vi "brick_break_game.vi"() -> (2 "Score":i32)   [LabVIEW 2014]
uses:
  <vilib>/Utility/miscctls.llb/LVPositionTypeDef.ctl
  <vilib>/Utility/miscctls.llb/LVBoundsTypeDef.ctl
panel:
  in  "ball":bool=TRUE
  in  "ball out":u32(colorbox)=16711680
  in  "ball in":u32(colorbox)=16711680
  out "xSpeedUp":bool
  out "ySpeedUp":bool
  in  "game string":string="Game Over"
  out "x speed up":string
  out "y speed up":string
  in  "Level":i32=1
  in  "game states":T1(ring)
  out "over":bool
  out "pass time":dbl
  in  "start":bool
  out "start timer":u32
  in  "ball init pos":cluster{i32, i32}
  out "brick status":bool[](array[boolean])
  out "bricks left":i32
  out "hit block":i32
  out "y hit detec":bool[][](array[boolean])
  out "y hitbox pos":i32[][](array[numeric])
  out "x hitbox pos":i32[][](array[numeric])
  out "ball size":i32
  in  "Brick 7":u32(colorbox)
  in  "Brick 6":u32(colorbox)
  in  "Brick 0":u32(colorbox)
  in  "Brick 5":u32(colorbox)
  in  "Brick 4":u32(colorbox)
  in  "Brick 3":u32(colorbox)
  in  "Brick 2":u32(colorbox)
  in  "Brick 1":u32(colorbox)
  out "brick pos":i32[][](array[numeric])
  in  "y scale":i32=2
  in  "x scale":i32=2
  in  "brick size":cluster{"width":i32, "hight":i32}={"width"=50, "hight"=20}
  in  "Slide":u8(slide)=100 scale=0.0..100.0
  out "x hit detec":bool[][](array[boolean])
  in  "backgound":T2={"width"=400, "hight"=300, "position"=[0, 0]}
  in  "background":u32(colorbox)=13816530
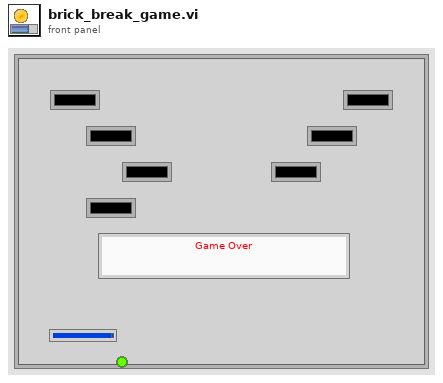
[diagram p1: front panel]
types:
  T1 = enum16{"Initialize", "Brick pos set Lv1", "Brick pos set Lv2", "Hitbox placement", "Level 1", "Level 2", "End"}
  T2 = cluster{"width":i32, "hight":i32, "position":i32[]}
  T3 = enum8{"Enabled", "Disabled", "Disabled and Grayed Out"}
  T4 = typedef "LVBoundsTypeDef.ctl" = cluster{"Width":u32, "Height":u32}
  T5 = typedef "LVPositionTypeDef.ctl" = cluster{"Left":i32, "Top":i32}
  T6 = typedef "eventvkey.ctl" = enum16{"ASCII", "Enter", "Return", "Shift", "Ctrl", "Alt", "Cmd", "Opt", "Caps", "NumLock", "Clear", "Break", "Up", "Down", "Left", "Right", "Insert", "Delete", "Home", "End", "PageUp", "PageDown", "Escape", "Help", "Pause", "ScrollLock", "F1", "F2", "F3", "F4", "F5", "F6", "F7", "F8", "F9", "F10", "F11", "F12", "F13", "F14", "F15", "F16", "F17", "F18", "F19", "F20", "F21", "F22", "F23", "F24", "Play", "VolumeUp", "VolumeDown", "Mute", "Two Byte Char"}
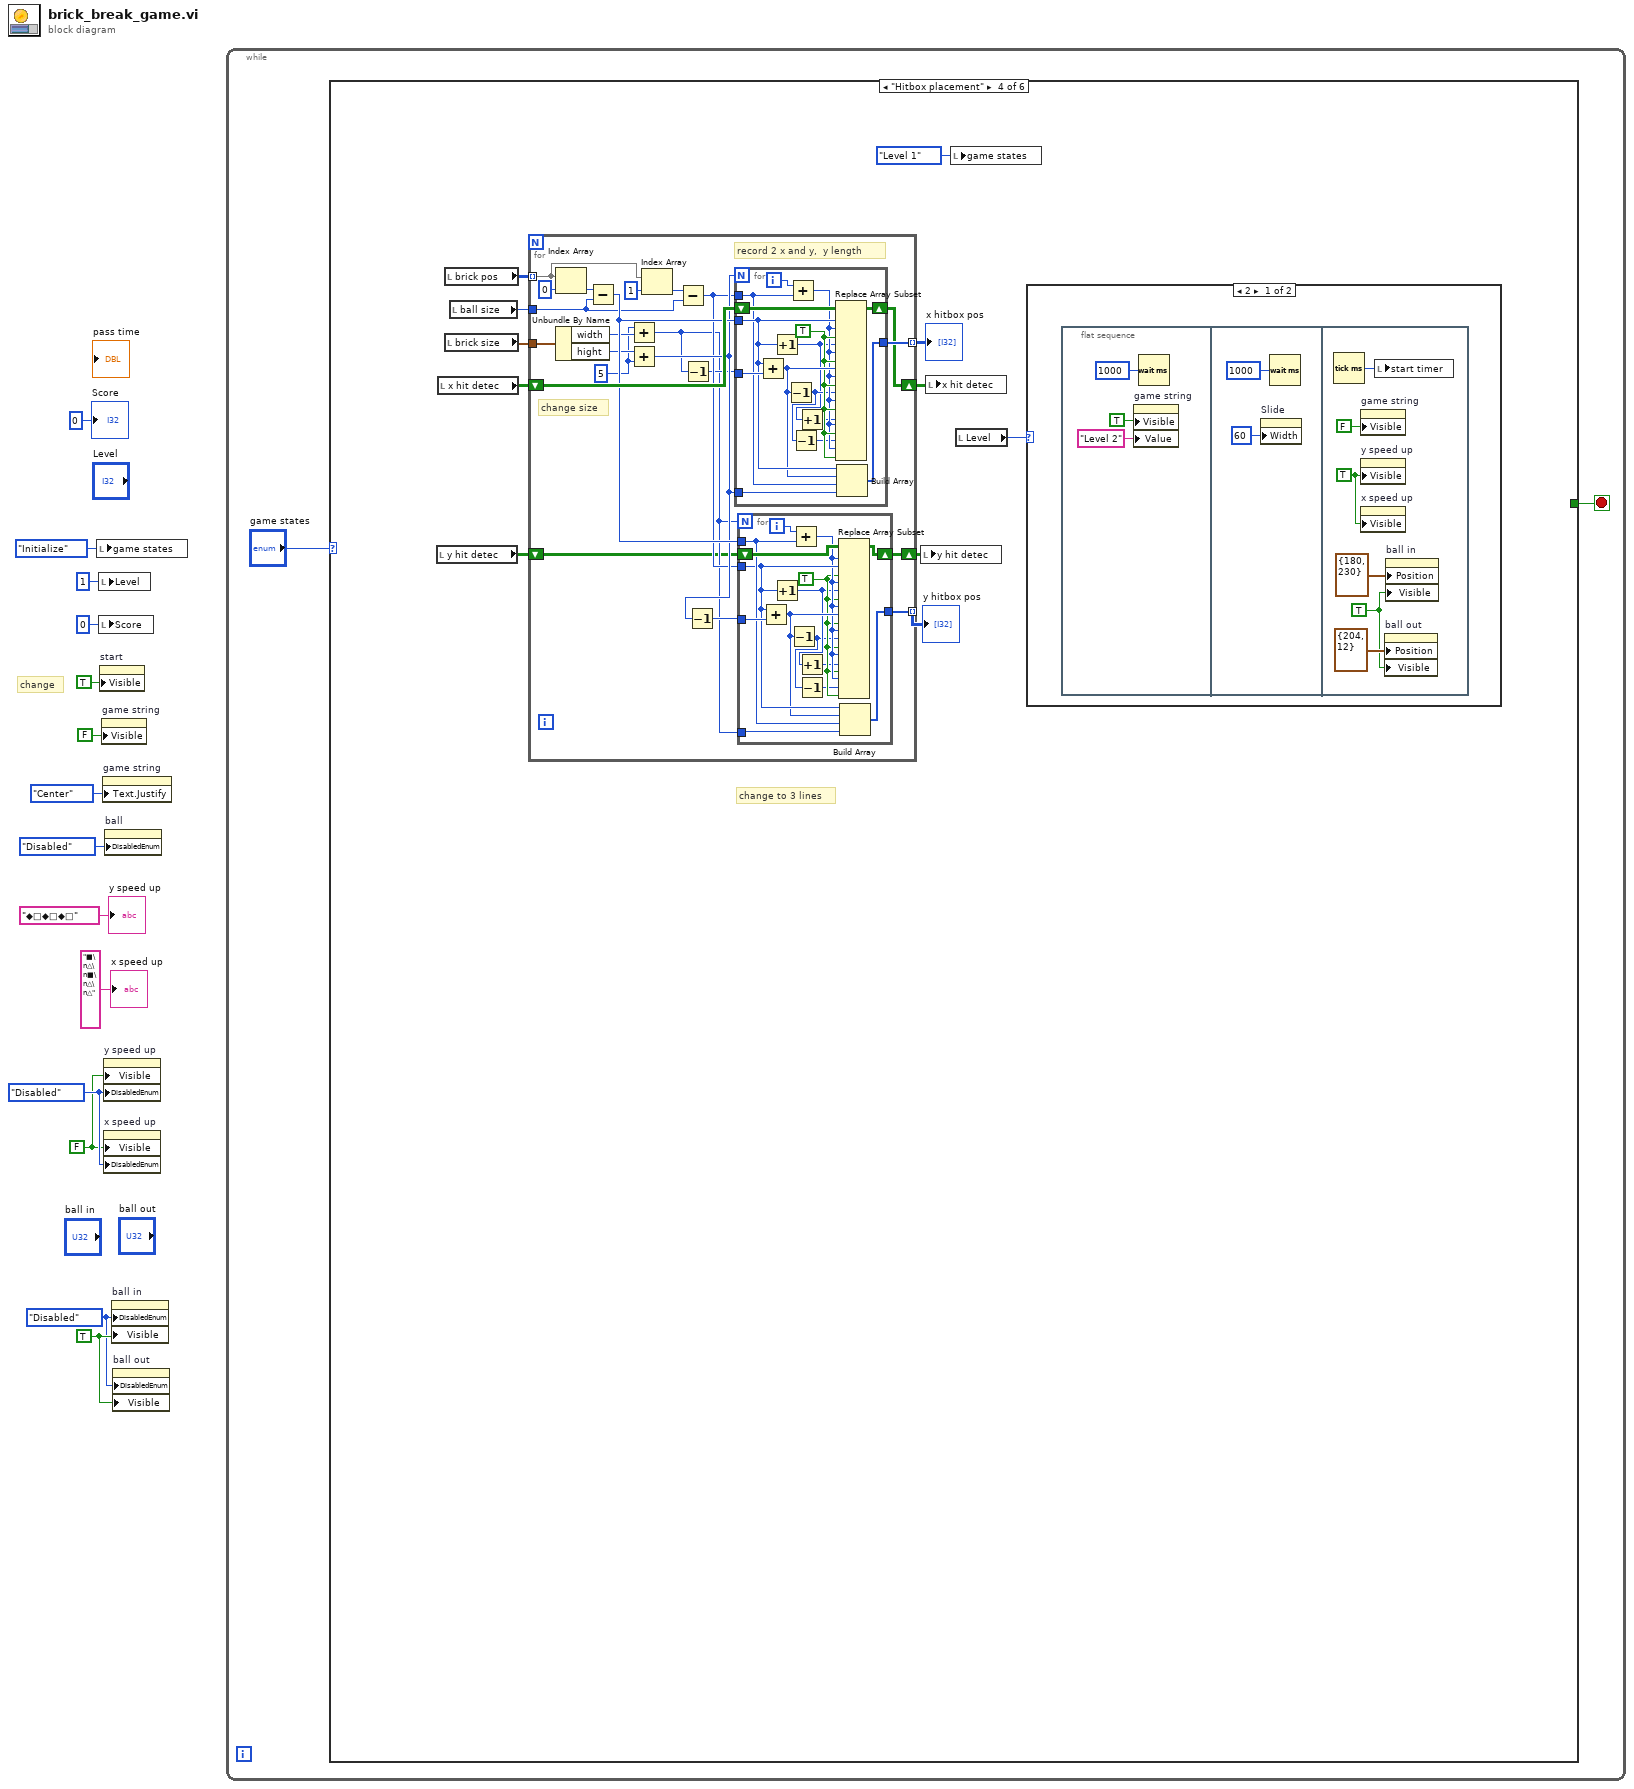
[diagram p0: block diagram]
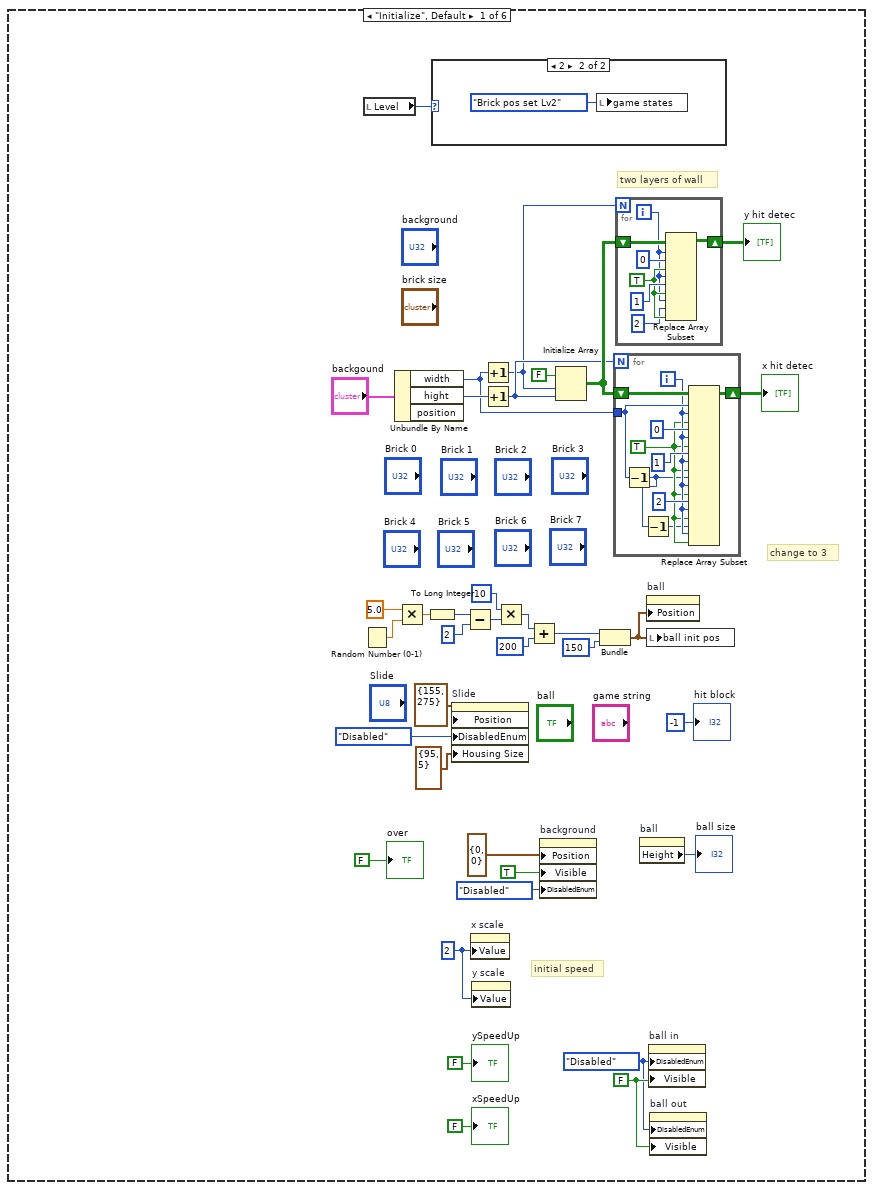
[diagram p2: hidden frame]
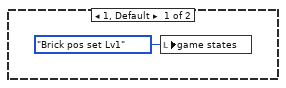
[diagram p3: hidden frame]
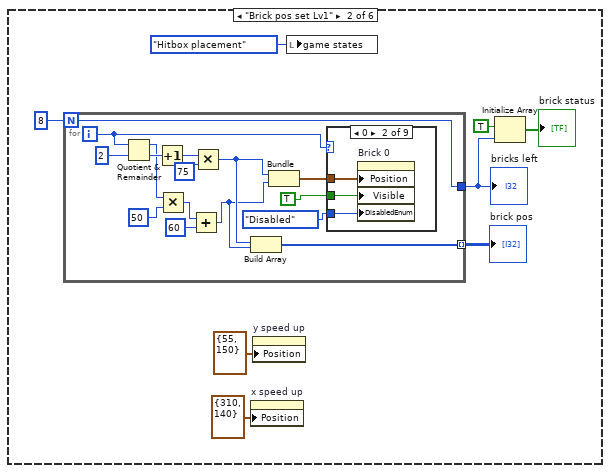
[diagram p4: hidden frame]
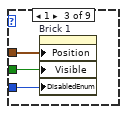
[diagram p6: hidden frame]
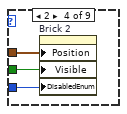
[diagram p7: hidden frame]
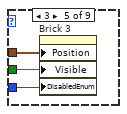
[diagram p8: hidden frame]
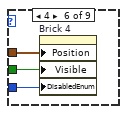
[diagram p9: hidden frame]
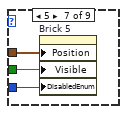
[diagram p10: hidden frame]
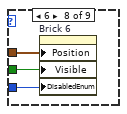
[diagram p11: hidden frame]
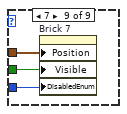
[diagram p12: hidden frame]
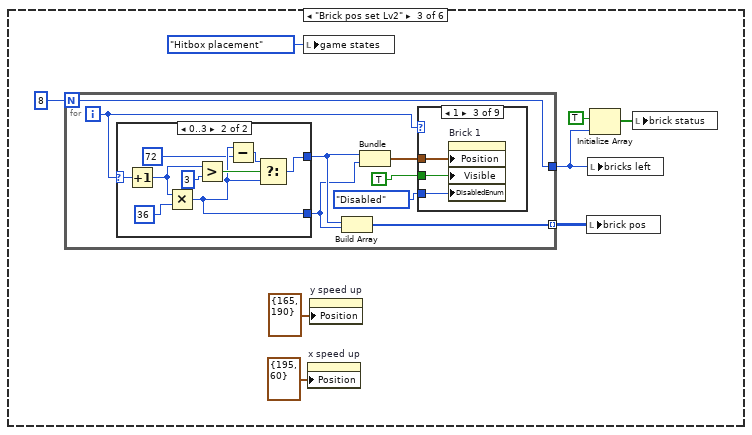
[diagram p13: hidden frame]
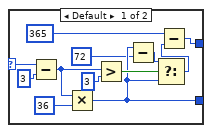
[diagram p14: hidden frame]
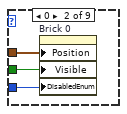
[diagram p16: hidden frame]
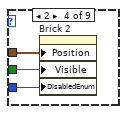
[diagram p17: hidden frame]
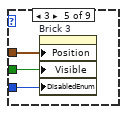
[diagram p18: hidden frame]
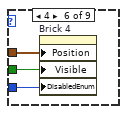
[diagram p19: hidden frame]
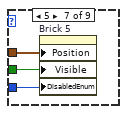
[diagram p20: hidden frame]
diagram:
  w2 = TRUE ("Visible")
  w1 = T3."Disabled" ("Disabled")
  w4 = T3."Disabled" ("Disabled")
  w3 = FALSE ("Visible")
  # "change"
  n1 = local write "game states"(T1."Initialize" ("game states")) -> ()
  n2 = local write "Level"(1 ("Level")) -> ()
  n3 = local write "Score"(0 ("Score")) -> ()
  n4 = property on="start" class="Bool"("Visible"=TRUE) -> ()  [unwired: 2 in, 2 out]
  n5 = property on="game string" class="Str"("Visible"=FALSE) -> ()  [unwired: 2 in, 2 out]
  n6 = property on="game string" class="Str"("Text.Justify"=enum16{"Left", "Center", "Right"}."Center" ("Text.Justification")) -> ()  [unwired: 2 in, 2 out]
  n7 = property on="y speed up" class="Str"("Visible"=w3, "DisabledEnum"=w4) -> ()  [unwired: 2 in, 2 out]
  n8 = property on="x speed up" class="Str"("Visible"=w3, "DisabledEnum"=w4) -> ()  [unwired: 2 in, 2 out]
  n9 = property on="ball" class="Bool (strict)"("DisabledEnum"=T3."Disabled" ("Disabled")) -> ()  [unwired: 2 in, 2 out]
  n10 = property on="ball in" class="ColBox"("DisabledEnum"=w1, "Visible"=w2) -> ()  [unwired: 2 in, 2 out]
  n11 = property on="ball out" class="ColBox"("DisabledEnum"=w1, "Visible"=w2) -> ()  [unwired: 2 in, 2 out]
  n12 = while {
    stop <- w15 stop-if-true
    n13 = case shown="\"Hitbox placement\"" "game states" {
      tunnel: [_ _ _ _ _ w845] -> w15
      frame "Initialize", Default {
        w18 = FALSE ("Visible")
        w17 = T3."Disabled" ("Disabled")
        w21 = 2 ("x scale")
        # "initial speed"
        # "change to 3"
        # "two layers of wall"
        n14 = Random Number (0-1)() -> (number: 0 to 1=w38:dbl)
        n15 = local read "Level"() -> (w23:i32)
        n16 = Unbundle By Name("backgound") -> ("width"=w46:i32, "hight"=w48:i32)  [unwired: 1 out]
        n17 = Multiply(x=5.0, y=w38) -> (x*y=w36:dbl)
        n18 = To Long Integer(number=w36) -> (32bit integer=w35:i32)
        n19 = case shown="2" w23 {
          frame 1, Default {
            n20 = local write "game states"(T1."Brick pos set Lv1" ("game states")) -> ()
          }
          frame 2 {
            n21 = local write "game states"(T1."Brick pos set Lv2" ("game states")) -> ()
          }
        }
        n22 = property on="Slide" class="Slide (strict)"("Position"=T5 {"Left"=155, "Top"=275}, "DisabledEnum"=T3."Disabled" ("Disabled"), "Housing Size"=T4 {"Width"=95, "Height"=5}) -> ()  [unwired: 2 in, 2 out]
        n23 = Subtract(x=w35, y=2) -> (x-y=w30:i32)
        n24 = property on="x scale" class="DigNum (strict)"("Value"=w21) -> ()  [unwired: 2 in, 2 out]
        n25 = property on="y scale" class="DigNum (strict)"("Value"=w21) -> ()  [unwired: 2 in, 2 out]
        n26 = Increment(x=w46) -> (x+1=w47:i32)
        n27 = Increment(x=w48) -> (x+1=w49:i32)
        n28 = Multiply(x=10 ("y"), y=w30) -> (x*y=w33:i32)
        n29 = Add(x=w33, y=200) -> (x+y=w31:i32)
        n30 = property on="background" class="ColBox"("Position"=T5 {"Left"=0, "Top"=0}, "Visible"=TRUE, "DisabledEnum"=T3."Disabled" ("Disabled")) -> ()  [unwired: 2 in, 2 out]
        n31 = Initialize Array(FALSE, w47, w49) -> (w50:bool[][])
        n32 = Bundle(w31, 150) -> (w40:cluster{i32, i32})  [unwired: 1 in]
        n33 = for {
          N: w49 -> [_]
          shift-right: [w70] -> w51
          shift-left: w50 -> [w71]
          tunnel: w46 -> [w68]
          i -> [w65]
          w64 = TRUE
          n34 = Decrement(x=w68) -> (x-1=w63:i32)
          n35 = Decrement(x=w63) -> (x-1=w62:i32)
          n36 = Replace Array Subset(array=w71, new element #1=w64, index (row) #1=w68, index (col) #1=w65, new element #2=w64, index (row) #2=0, index (col) #2=w65, new element #3=w64, index (row) #3=1 ("disabled index (row)"), index (col) #3=w65, new element #4=w64, index (row) #4=w63, index (col) #4=w65, new element #5=w64, index (row) #5=2, index (col) #5=w65, new element #6=w64, index (row) #6=w62, index (col) #6=w65) -> (w70:bool[][])
        }
        "x hit detec" <- w51
        n37 = for {
          N: w47 -> [_]
          shift-right: [w60] -> w52
          shift-left: w50 -> [w61]
          i -> [w56]
          w57 = TRUE
          n38 = Replace Array Subset(array=w61, new element #1=w57, index (row) #1=w56, index (col) #1=0 ("index (col)"), new element #2=w57, index (row) #2=w56, index (col) #2=1 ("disabled index (col)"), new element #3=w57, index (row) #3=w56, index (col) #3=2) -> (w60:bool[][])
        }
        "y hit detec" <- w52
        n39 = property on="ball" class="Bool (strict)"() -> ("Height"=→"ball size":u32)  [unwired: 2 in, 2 out]
        n40 = property on="ball" class="Bool (strict)"("Position"=w40) -> ()  [unwired: 2 in, 2 out]
        n41 = local write "ball init pos"(w40) -> ()
        n42 = property on="ball in" class="ColBox"("DisabledEnum"=w17, "Visible"=w18) -> ()  [unwired: 2 in, 2 out]
        n43 = property on="ball out" class="ColBox"("DisabledEnum"=w17, "Visible"=w18) -> ()  [unwired: 2 in, 2 out]
        "hit block" <- -1 ("hit block")
        "over" <- FALSE ("over")
        "ySpeedUp" <- FALSE ("ySpeedUp")
        "xSpeedUp" <- FALSE ("xSpeedUp")
      }
      frame "Brick pos set Lv1" {
        n44 = for {
          N: 8 -> [w80]
          tunnel: [w86] -> w78 mode=indexing
          tunnel: [w80] -> w76
          i -> [w81]
          n45 = Quotient & Remainder(x=w81, y=2) -> (x-y*floor(x/y)=w88:i32, floor(x/y)=w93:i32)
          n46 = Increment(x=w93) -> (x+1=w92:i32)
          n47 = Multiply(x=w88, y=50) -> (x*y=w85:i32)
          n48 = Add(x=w85, y=60) -> (x+y=w84:i32)
          n49 = Multiply(x=w92, y=75) -> (x*y=w87:i32)
          n50 = Build Array(w87, w84) -> (w86:i32[])
          n51 = Bundle(w87, w84) -> (w89:cluster{i32, i32})  [unwired: 1 in]
          n52 = case shown="0" w81 {
            tunnel: TRUE -> [_ w98 w101 w104 w107 w110 w113 w115 w119]
            tunnel: w89 -> [_ w97 w100 w103 w106 w109 w112 w116 w118]
            tunnel: T3."Disabled" ("Disabled") -> [_ w96 w99 w102 w105 w108 w111 w114 w117]
            frame Default {
            }
            frame 0 {
              n53 = property on="Brick 0" class="ColBox"("Position"=w97, "Visible"=w98, "DisabledEnum"=w96) -> ()  [unwired: 2 in, 2 out]
            }
            frame 1 {
              n54 = property on="Brick 1" class="ColBox"("Position"=w100, "Visible"=w101, "DisabledEnum"=w99) -> ()  [unwired: 2 in, 2 out]
            }
            frame 2 {
              n55 = property on="Brick 2" class="ColBox"("Position"=w103, "Visible"=w104, "DisabledEnum"=w102) -> ()  [unwired: 2 in, 2 out]
            }
            frame 3 {
              n56 = property on="Brick 3" class="ColBox"("Position"=w106, "Visible"=w107, "DisabledEnum"=w105) -> ()  [unwired: 2 in, 2 out]
            }
            frame 4 {
              n57 = property on="Brick 4" class="ColBox"("Position"=w109, "Visible"=w110, "DisabledEnum"=w108) -> ()  [unwired: 2 in, 2 out]
            }
            frame 5 {
              n58 = property on="Brick 5" class="ColBox"("Position"=w112, "Visible"=w113, "DisabledEnum"=w111) -> ()  [unwired: 2 in, 2 out]
            }
            frame 6 {
              n59 = property on="Brick 6" class="ColBox"("Position"=w116, "Visible"=w115, "DisabledEnum"=w114) -> ()  [unwired: 2 in, 2 out]
            }
            frame 7 {
              n60 = property on="Brick 7" class="ColBox"("Position"=w118, "Visible"=w119, "DisabledEnum"=w117) -> ()  [unwired: 2 in, 2 out]
            }
          }
        }
        "brick pos" <- w78
        "bricks left" <- w76
        n61 = property on="x speed up" class="Str"("Position"=T5 {"Left"=310, "Top"=140}) -> ()  [unwired: 2 in, 2 out]
        n62 = property on="y speed up" class="Str"("Position"=T5 {"Left"=55, "Top"=150}) -> ()  [unwired: 2 in, 2 out]
        n63 = local write "game states"(T1."Hitbox placement" ("game states")) -> ()
        n64 = Initialize Array(TRUE, w76) -> (→"brick status":bool[])
      }
      frame "Brick pos set Lv2" {
        n65 = for {
          N: 8 -> [w131]
          tunnel: [w133] -> w123 mode=indexing
          tunnel: [w131] -> w122
          i -> [w128]
          n66 = case shown="0..3" w128 {
            selector: w128 -> [w147 w156]
            tunnel: [w137 w149] -> w130
            tunnel: [w140 w152] -> w129
            frame Default {
              n67 = Subtract(x=w147, y=3) -> (x-y=w141:i32)
              n68 = Multiply(x=w141, y=36) -> (x*y=w140:i32)
              n69 = Greater?(x=w141, y=3) -> (0:w143:bool)
              n70 = Subtract(x=w140, y=72) -> (x-y=w142:i32)
              n71 = Select(t=w142, s=w143, f=w140) -> (s? t:f=w138:i32)
              n72 = Subtract(x=365, y=w138) -> (x-y=w137:i32)
            }
            frame 0..3 {
              n73 = Increment(x=w156) -> (x+1=w155:i32)
              n74 = Multiply(x=w155, y=36) -> (x*y=w152:i32)
              n75 = Greater?(x=w155, y=3) -> (0:w153:bool)
              n76 = Subtract(x=w152, y=72) -> (x-y=w150:i32)
              n77 = Select(t=w150, s=w153, f=w152) -> (s? t:f=w149:i32)
            }
          }
          n78 = Build Array(w130, w129) -> (w133:i32[])
          n79 = Bundle(w130, w129) -> (w134:cluster{i32, i32})  [unwired: 1 in]
          n80 = case shown="1" w128 {
            tunnel: TRUE -> [_ w159 w162 w165 w168 w171 w174 w176 w180]
            tunnel: w134 -> [_ w158 w161 w164 w167 w170 w173 w177 w179]
            tunnel: T3."Disabled" ("Disabled") -> [_ w157 w160 w163 w166 w169 w172 w175 w178]
            frame Default {
            }
            frame 0 {
              n81 = property on="Brick 0" class="ColBox"("Position"=w158, "Visible"=w159, "DisabledEnum"=w157) -> ()  [unwired: 2 in, 2 out]
            }
            frame 1 {
              n82 = property on="Brick 1" class="ColBox"("Position"=w161, "Visible"=w162, "DisabledEnum"=w160) -> ()  [unwired: 2 in, 2 out]
            }
            frame 2 {
              n83 = property on="Brick 2" class="ColBox"("Position"=w164, "Visible"=w165, "DisabledEnum"=w163) -> ()  [unwired: 2 in, 2 out]
            }
            frame 3 {
              n84 = property on="Brick 3" class="ColBox"("Position"=w167, "Visible"=w168, "DisabledEnum"=w166) -> ()  [unwired: 2 in, 2 out]
            }
            frame 4 {
              n85 = property on="Brick 4" class="ColBox"("Position"=w170, "Visible"=w171, "DisabledEnum"=w169) -> ()  [unwired: 2 in, 2 out]
            }
            frame 5 {
              n86 = property on="Brick 5" class="ColBox"("Position"=w173, "Visible"=w174, "DisabledEnum"=w172) -> ()  [unwired: 2 in, 2 out]
            }
            frame 6 {
              n87 = property on="Brick 6" class="ColBox"("Position"=w177, "Visible"=w176, "DisabledEnum"=w175) -> ()  [unwired: 2 in, 2 out]
            }
            frame 7 {
              n88 = property on="Brick 7" class="ColBox"("Position"=w179, "Visible"=w180, "DisabledEnum"=w178) -> ()  [unwired: 2 in, 2 out]
            }
          }
        }
        n89 = local write "game states"(T1."Hitbox placement" ("game states")) -> ()
        n90 = property on="x speed up" class="Str"("Position"=T5 {"Left"=195, "Top"=60}) -> ()  [unwired: 2 in, 2 out]
        n91 = property on="y speed up" class="Str"("Position"=T5 {"Left"=165, "Top"=190}) -> ()  [unwired: 2 in, 2 out]
        n92 = local write "brick pos"(w123) -> ()
        n93 = local write "bricks left"(w122) -> ()
        n94 = Initialize Array(TRUE, w122) -> (w125:bool[])
        n95 = local write "brick status"(w125) -> ()
      }
      frame "Hitbox placement" {
        # "change to 3 lines"
        n96 = local read "y hit detec"() -> (w190:bool[][])
        n97 = local read "x hit detec"() -> (w184:bool[][])
        n98 = local read "brick pos"() -> (w183:i32[][])
        n99 = local read "brick size"() -> (w185:cluster{"width":i32, "hight":i32})
        n100 = local read "ball size"() -> (w186:i32)
        n101 = for {
          tunnel: w183 -> [w236] mode=indexing
          tunnel: w185 -> [w239]
          tunnel: w186 -> [w227]
          shift-right: [w221] -> w187
          shift-left: w184 -> [w233]
          tunnel: [w232] -> w188 mode=indexing
          tunnel: [w230] -> w189 mode=indexing
          shift-right: [w219] -> w191
          shift-left: w190 -> [w220]
          w218 = 5
          # "change size"
          # "record 2 x and y,  y length"
          n102 = Index Array(array=w236, index=0) -> (element=w235:i32)
          n103 = Unbundle By Name(w239) -> ("width"=w229:i32, "hight"=w228:i32)
          n104 = Subtract(x=w235, y=w227) -> (x-y=w231:i32)
          n105 = Add(x=w218, y=w229) -> (x+y=w222:i32)
          n106 = Add(x=w228, y=w218) -> (x+y=w226:i32)
          n107 = Index Array(array=w236, index=1) -> (element=w234:i32)
          n108 = Subtract(x=w234, y=w227) -> (x-y=w224:i32)
          n109 = Decrement(x=w222) -> (x-1=w223:i32)
          n110 = Decrement(x=w226) -> (x-1=w225:i32)
          n111 = for {
            N: w226 -> [_]
            tunnel: w231 -> [w265]
            tunnel: w224 -> [w261]
            tunnel: w223 -> [w267]
            shift-right: [w266] -> w221
            shift-left: w233 -> [w269]
            tunnel: [w264] -> w232
            tunnel: w226 -> [w262]
            i -> [w268]
            w260 = TRUE
            n112 = Add(x=w265, y=w267) -> (x+y=w263:i32)
            n113 = Increment(x=w265) -> (x+1=w255:i32)
            n114 = Decrement(x=w263) -> (x-1=w257:i32)
            n115 = Add(x=w268, y=w261) -> (x+y=w259:i32)
            n116 = Decrement(x=w257) -> (x-1=w258:i32)
            n117 = Increment(x=w255) -> (x+1=w256:i32)
            n118 = Replace Array Subset(array=w269, new element #1=w260, index (row) #1=w265, index (col) #1=w259, new element #2=w260, index (row) #2=w255, index (col) #2=w259, new element #3=w260, index (row) #3=w263, index (col) #3=w259, new element #4=w260, index (row) #4=w257, index (col) #4=w259, new element #5=w260, index (row) #5=w256, index (col) #5=w259, new element #6=w260, index (row) #6=w258, index (col) #6=w259) -> (w266:bool[][])
            n119 = Build Array(w265, w263, w261, w262) -> (w264:i32[])
          }
          n120 = for {
            N: w222 -> [_]
            tunnel: w224 -> [w247]
            tunnel: w231 -> [w248]
            tunnel: w225 -> [w252]
            shift-right: [w251] -> w219
            shift-left: w220 -> [w254]
            tunnel: [w250] -> w230
            tunnel: w222 -> [w249]
            i -> [w253]
            w244 = TRUE
            n121 = Add(x=w247, y=w252) -> (x+y=w246:i32)
            n122 = Increment(x=w247) -> (x+1=w242:i32)
            n123 = Decrement(x=w246) -> (x-1=w240:i32)
            n124 = Add(x=w253, y=w248) -> (x+y=w245:i32)
            n125 = Increment(x=w242) -> (x+1=w243:i32)
            n126 = Decrement(x=w240) -> (x-1=w241:i32)
            n127 = Replace Array Subset(array=w254, new element #1=w244, index (row) #1=w245, index (col) #1=w247, new element #2=w244, index (row) #2=w245, index (col) #2=w242, new element #3=w244, index (row) #3=w245, index (col) #3=w246, new element #4=w244, index (row) #4=w245, index (col) #4=w240, new element #5=w244, index (row) #5=w245, index (col) #5=w243, new element #6=w244, index (row) #6=w245, index (col) #6=w241) -> (w251:bool[][])
            n128 = Build Array(w247, w246, w248, w249) -> (w250:i32[])
          }
        }
        "x hitbox pos" <- w188
        "y hitbox pos" <- w189
        n129 = local write "y hit detec"(w191) -> ()
        n130 = local write "x hit detec"(w187) -> ()
        n131 = local write "game states"(T1."Level 1" ("game states")) -> ()
        n132 = local read "Level"() -> (w182:i32)
        n133 = case shown="2" w182 {
          frame 2 {
            n134 = flat-sequence {
              frame #0 {
                n135 = property on="game string" class="Str"("Visible"=TRUE, "Value"="Level 2" ("game over")) -> ()  [unwired: 2 in, 2 out]
                n136 = Wait (ms)(milliseconds to wait=u32 1000) -> ()  [unwired: 1 out]
              }
              frame #1 {
                n137 = property on="Slide" class="Slide (strict)"("Width"=u32 60 ("Housing Size:Width")) -> ()  [unwired: 2 in, 2 out]
                n138 = Wait (ms)(milliseconds to wait=u32 1000) -> ()  [unwired: 1 out]
              }
              frame #2 {
                w198 = TRUE
                w200 = TRUE ("Visible")
                n139 = Tick Count (ms)() -> (millisecond timer value=w201:u32)
                n140 = property on="game string" class="Str"("Visible"=FALSE) -> ()  [unwired: 2 in, 2 out]
                n141 = property on="y speed up" class="Str"("Visible"=w200) -> ()  [unwired: 2 in, 2 out]
                n142 = property on="x speed up" class="Str"("Visible"=w200) -> ()  [unwired: 2 in, 2 out]
                n143 = local write "start timer"(w201) -> ()
                n144 = property on="ball out" class="ColBox"("Position"=T5 {"Left"=204, "Top"=12}, "Visible"=w198) -> ()  [unwired: 2 in, 2 out]
                n145 = property on="ball in" class="ColBox"("Position"=T5 {"Left"=180, "Top"=230}, "Visible"=w198) -> ()  [unwired: 2 in, 2 out]
              }
            }
          }
          frame 1, Default {
            n146 = while {
              stop <- w203 stop-if-true
              n147 = case shown="True" "start" {
                selector: "start" -> [w206 w207]
                tunnel: [w206 w207] -> w203
                frame False {
                }
                frame True {
                  n148 = flat-sequence {
                    frame #0 {
                      n149 = property on="start" class="Bool"("Visible"=FALSE) -> ()  [unwired: 2 in, 2 out]
                      n150 = property on="game string" class="Str"("Visible"=TRUE, "Value"="Level 1" ("game over")) -> ()  [unwired: 2 in, 2 out]
                      n151 = Wait (ms)(milliseconds to wait=u32 1000) -> ()  [unwired: 1 out]
                    }
                    frame #1 {
                      w213 = TRUE
                      w215 = TRUE ("Visible")
                      n152 = Tick Count (ms)() -> (millisecond timer value=→"start timer":u32)
                      n153 = property on="game string" class="Str"("Visible"=FALSE) -> ()  [unwired: 2 in, 2 out]
                      n154 = property on="ball out" class="ColBox"("Position"=T5 {"Left"=204, "Top"=12}, "Visible"=w213) -> ()  [unwired: 2 in, 2 out]
                      n155 = property on="ball in" class="ColBox"("Position"=T5 {"Left"=180, "Top"=230}, "Visible"=w213) -> ()  [unwired: 2 in, 2 out]
                      n156 = property on="y speed up" class="Str"("Visible"=w215) -> ()  [unwired: 2 in, 2 out]
                      n157 = property on="x speed up" class="Str"("Visible"=w215) -> ()  [unwired: 2 in, 2 out]
                    }
                  }
                }
              }
              n158 = Wait Until Next ms Multiple(millisecond multiple=u32 100 ("milliseconds to wait")) -> ()  [unwired: 1 out]
            }
          }
        }
      }
      frame "Level 1" {
        # "red hole move"
        # "speed up"
        # "delete bricks"
        # "ball movements"
        # "control slide"
        n159 = local read "Level"() -> (w273:i32)
        n160 = while {
          stop <- w709 stop-if-true
          n161 = event shown="[0] \"hit block\": Value Change" {
            selector: _ -> [_ _]
            dyn-events: _ -> [_ _]
            timeout: _ -> [_ _]
            tunnel: [w713 w776] -> w709
            event "hit block": Value Change {
              n162 = event-data() -> ("NewVal"=w711:i32)  [unwired: 1 in]
              n163 = local read "brick status"() -> (w712:bool[])
              n164 = Index Array(array=w712, index=w711) -> (element=w710:bool)
              n165 = case shown="True" w710 {
                tunnel: w711 -> [_ w717]
                tunnel: [FALSE w720] -> w713
                frame False {
                }
                frame True {
                  w736 = 3 ("index")
                  w737 = 2 ("index")
                  w738 = 1 ("index")
                  w739 = 0 ("index")
                  # "change to 3"
                  n166 = local read "brick status"() -> (w718:bool[])
                  n167 = local read "x hitbox pos"() -> (w743:i32[][])
                  n168 = local read "y hitbox pos"() -> (w742:i32[][])
                  n169 = local read "bricks left"() -> (w722:i32)
                  n170 = local write "hit block"(-1 ("hit block")) -> ()
                  n171 = Decrement(x=w722) -> (x-1=w721:i32)
                  n172 = Replace Array Subset(array=w718, new element=FALSE ("new element/subarray"), index=w717) -> (w715:bool[])
                  n173 = case shown="7" w717 {
                    tunnel: FALSE -> [_ w744 w745 w746 w747 w748 w749 w750 w751]
                    frame Default {
                    }
                    frame 0 {
                      n174 = property on="Brick 0" class="ColBox"("Visible"=w744) -> ()  [unwired: 2 in, 2 out]
                    }
                    frame 1 {
                      n175 = property on="Brick 1" class="ColBox"("Visible"=w745) -> ()  [unwired: 2 in, 2 out]
                    }
                    frame 2 {
                      n176 = property on="Brick 2" class="ColBox"("Visible"=w746) -> ()  [unwired: 2 in, 2 out]
                    }
                    frame 3 {
                      n177 = property on="Brick 3" class="ColBox"("Visible"=w747) -> ()  [unwired: 2 in, 2 out]
                    }
                    frame 4 {
                      n178 = property on="Brick 4" class="ColBox"("Visible"=w748) -> ()  [unwired: 2 in, 2 out]
                    }
                    frame 5 {
                      n179 = property on="Brick 5" class="ColBox"("Visible"=w749) -> ()  [unwired: 2 in, 2 out]
                    }
                    frame 6 {
                      n180 = property on="Brick 6" class="ColBox"("Visible"=w750) -> ()  [unwired: 2 in, 2 out]
                    }
                    frame 7 {
                      n181 = property on="Brick 7" class="ColBox"("Visible"=w751) -> ()  [unwired: 2 in, 2 out]
                    }
                  }
                  n182 = Index Array(array=w743, index (row)=w717) -> (element=w741:i32[])  [unwired: 1 in]
                  n183 = Index Array(array=w742, index (row)=w717) -> (element=w740:i32[])  [unwired: 1 in]
                  n184 = Equal To 0?(x=w721) -> (x = 0?=w720:bool)
                  n185 = property on="bricks left" class="DigNum (strict)"("Val(Sgnl)"=w721) -> ()  [unwired: 2 in, 2 out]
                  n186 = local write "brick status"(w715) -> ()
                  n187 = Index Array(array=w741, index #1=w739, index #2=w738, index #3=w737, index #4=w736) -> (element #1=w733:i32, element #2=w732:i32, element #3=w731:i32, element #4=w734:i32)
                  n188 = Index Array(array=w740, index #1=w739, index #2=w738, index #3=w737, index #4=w736) -> (element #1=w727:i32, element #2=w726:i32, element #3=w725:i32, element #4=w728:i32)
                  n189 = local read "y hit detec"() -> (w729:bool[][])
                  n190 = local read "x hit detec"() -> (w735:bool[][])
                  n191 = for {
                    N: w734 -> [_]
                    shift-right: [w774] -> w730
                    shift-left: w735 -> [w775]
                    tunnel: w733 -> [w773]
                    tunnel: w732 -> [w772]
                    tunnel: w731 -> [w770]
                    i -> [w771]
                    w769 = FALSE
                    n192 = Add(x=w770, y=w771) -> (x+y=w768:i32)
                    n193 = Increment(x=w773) -> (x+1=w767:i32)
                    n194 = Decrement(x=w772) -> (x-1=w765:i32)
                    n195 = Increment(x=w767) -> (x+1=w766:i32)
                    n196 = Decrement(x=w765) -> (x-1=w764:i32)
                    n197 = Replace Array Subset(array=w775, new element #1=w769, index (row) #1=w773, index (col) #1=w768, new element #2=w769, index (row) #2=w767, index (col) #2=w768, new element #3=w769, index (row) #3=w772, index (col) #3=w768, new element #4=w769, index (row) #4=w765, index (col) #4=w768, new element #5=w769, index (row) #5=w766, index (col) #5=w768, new element #6=w769, index (row) #6=w764, index (col) #6=w768) -> (w774:bool[][])
                  }
                  n198 = for {
                    N: w728 -> [_]
                    shift-right: [w762] -> w724
                    shift-left: w729 -> [w763]
                    tunnel: w727 -> [w759]
                    tunnel: w726 -> [w758]
                    tunnel: w725 -> [w760]
                    i -> [w761]
                    w757 = FALSE
                    n199 = Add(x=w760, y=w761) -> (x+y=w756:i32)
                    n200 = Increment(x=w759) -> (x+1=w755:i32)
                    n201 = Decrement(x=w758) -> (x-1=w753:i32)
                    n202 = Increment(x=w755) -> (x+1=w754:i32)
                    n203 = Decrement(x=w753) -> (x-1=w752:i32)
                    n204 = Replace Array Subset(array=w763, new element #1=w757, index (row) #1=w756, index (col) #1=w759, new element #2=w757, index (row) #2=w756, index (col) #2=w755, new element #3=w757, index (row) #3=w756, index (col) #3=w758, new element #4=w757, index (row) #4=w756, index (col) #4=w753, new element #5=w757, index (row) #5=w756, index (col) #5=w754, new element #6=w757, index (row) #6=w756, index (col) #6=w752) -> (w762:bool[][])
                  }
                  n205 = local write "x hit detec"(w730) -> ()
                  n206 = local write "y hit detec"(w724) -> ()
                }
              }
            }
            event "over": Value Change {
              n207 = event-data() -> ("NewVal"=w776:bool)  [unwired: 1 in]
            }
          }
        }
        n208 = case shown="1, Default" w273 {
          frame 1, Default {
            w337 = FALSE
            n209 = Random Number (0-1)() -> (number: 0 to 1=w340:dbl)
            n210 = To Long Integer(number=w340) -> (32bit integer=w339:i32)
            n211 = case shown="0, Default" w339 {
              selector: w339 -> [_ w346]
              tunnel: [-1 w346] -> w344
              frame 0, Default {
              }
              frame 1 {
              }
            }
            n212 = Unbundle("ball init pos") -> (w342:i32, w343:i32)
            n213 = while {
              shift-right: [w348] -> _
              shift-left: w342 -> [w354]
              shift-right: [w347] -> _
              shift-left: w343 -> [w355]
              shift-right: [w402] -> _
              shift-left: w344 -> [w407]
              shift-right: [w392] -> _
              shift-left: 1 -> [w405]
              shift-right: [w360] -> _
              shift-left: w337 -> [w363]
              shift-right: [w357] -> _
              shift-left: w337 -> [w362]
              stop <- w394 stop-if-true
              w366 = 45
              w380 = 45
              # "init value set"
              n214 = flat-sequence {
                tunnel: w354 -> [w416]
                tunnel: w355 -> [w415]
                tunnel: [w414] -> w350
                tunnel: [w413] -> w353
                tunnel: [w412] -> w351
                frame #0 {
                  # "x"
                  # "y"
                  n215 = property on="ball in" class="ColBox"() -> ("Bounds"=w438:T4)  [unwired: 2 in, 2 out]
                  n216 = property on="ball in" class="ColBox"() -> ("Position"=w437:T5)  [unwired: 2 in, 2 out]
                  n217 = Unbundle(w438) -> ("Width"=w421:u32, "Height"=w422:u32)
                  n218 = Unbundle(w437) -> ("Left"=w430:i32, "Top"=w428:i32)
                  n219 = To Quad Integer(1:w422) -> (0:w419:i64)
                  n220 = To Quad Integer(1:w421) -> (0:w420:i64)
                  n221 = Subtract(x=w420, y=u32 10) -> (x-y=w427:i64)
                  n222 = Subtract(x=w419, y=i64 10) -> (x-y=w426:i64)
                  n223 = Subtract(x=w415, y=w428) -> (x-y=w425:i32)
                  n224 = Subtract(x=w416, y=w430) -> (x-y=w429:i32)
                  n225 = Greater?(x=w429, y=-1) -> (0:w435:bool)
                  n226 = Less?(x=w429, y=w427) -> (x < y?=w436:bool)
                  n227 = Greater Or Equal?(x=w425, y=-1) -> (x >= y?=w432:bool)
                  n228 = Less Or Equal?(x=w425, y=w426) -> (x <= y?=w431:bool)
                  n229 = And(x=w435, y=w436) -> (x .and. y?=w434:bool)
                  n230 = And(x=w432, y=w431) -> (x .and. y?=w433:bool)
                  n231 = And(x=w434, y=w433) -> (x .and. y?=w417:bool)
                  n232 = case shown="True" w417 {
                    selector: w417 -> [w439 w442]
                    tunnel: w416 -> [w441 _]
                    tunnel: w415 -> [w440 _]
                    tunnel: [w441 w444] -> w414
                    tunnel: [w440 w443] -> w413
                    tunnel: [w439 w442] -> w412
                    frame False {
                    }
                    frame True {
                      w448 = 2.0 ("y")
                      w455 = 3 ("x")
                      n233 = property on="ball out" class="ColBox"() -> ("Position"=w458:T5)  [unwired: 2 in, 2 out]
                      n234 = Random Number (0-1)() -> (number: 0 to 1=w446:dbl)
                      n235 = Random Number (0-1)() -> (number: 0 to 1=w447:dbl)
                      n236 = Multiply(x=w446, y=w448) -> (x*y=w449:dbl)
                      n237 = Multiply(x=w447, y=w448) -> (x*y=w450:dbl)
                      n238 = Unbundle(w458) -> ("Left"=w457:i32, "Top"=w456:i32)
                      n239 = To Long Integer(number=w449) -> (32bit integer=w452:i32)
                      n240 = To Long Integer(number=w450) -> (32bit integer=w451:i32)
                      n241 = Increment(x=w452) -> (x+1=w453:i32)
                      n242 = Increment(x=w451) -> (x+1=w454:i32)
                      n243 = Add(x=w455, y=w457) -> (x+y=w444:i32)
                      n244 = Add(x=w456, y=w455) -> (x+y=w443:i32)
                      n245 = property on="y scale" class="DigNum (strict)"("Value"=w453) -> ()  [unwired: 2 in, 2 out]
                      n246 = property on="x scale" class="DigNum (strict)"("Value"=w454) -> ()  [unwired: 2 in, 2 out]
                      n247 = Bundle(w444, w443) -> (w459:cluster{i32, i32})  [unwired: 1 in]
                      n248 = property on="ball" class="Bool (strict)"("Position"=w459) -> ()  [unwired: 2 in, 2 out]
                      n249 = Wait (ms)(milliseconds to wait=u32 300) -> ()  [unwired: 1 out]
                    }
                  }
                }
              }
              n250 = local read "x hit detec"() -> (w410:bool[][])
              n251 = local read "y hit detec"() -> (w409:bool[][])
              n252 = Not(x=w363) -> (.not. x?=w359:bool)
              n253 = Not(x=w362) -> (.not. x?=w356:bool)
              n254 = Index Array(array=w410, index (row)=w354, index (col)=w355) -> (element=w408:bool)
              n255 = Index Array(array=w409, index (row)=w354, index (col)=w355) -> (element=w406:bool)
              n256 = case shown="True" w408 {
                tunnel: w407 -> [w505 w510]
                tunnel: [w505 w508] -> w402
                tunnel: w354 -> [_ w507]
                tunnel: w355 -> [_ w506]
                frame False {
                }
                frame True {
                  n257 = Multiply(x=-1, y=w510) -> (x*y=w508:i32)
                  n258 = case shown="60..130" w507 {
                    tunnel: w506 -> [_ w511 w514 w517 w520]
                    frame 0, Default {
                    }
                    frame 60..130 {
                      n259 = case shown="45..85" w511 {
                        frame 0, Default {
                        }
                        frame 45..85 {
                          n260 = property on="hit block" class="DigNum (strict)"("Val(Sgnl)"=0 ("hit block")) -> ()  [unwired: 2 in, 2 out]
                        }
                        frame 95..135 {
                          n261 = property on="hit block" class="DigNum (strict)"("Val(Sgnl)"=1 ("hit block")) -> ()  [unwired: 2 in, 2 out]
                        }
                      }
                    }
                    frame 135..205 {
                      n262 = case shown="45..85" w514 {
                        frame 0, Default {
                        }
                        frame 45..85 {
                          n263 = property on="hit block" class="DigNum (strict)"("Val(Sgnl)"=2 ("hit block")) -> ()  [unwired: 2 in, 2 out]
                        }
                        frame 95..135 {
                          n264 = property on="hit block" class="DigNum (strict)"("Val(Sgnl)"=3 ("hit block")) -> ()  [unwired: 2 in, 2 out]
                        }
                      }
                    }
                    frame 210..280 {
                      n265 = case shown="45..85" w517 {
                        frame 0, Default {
                        }
                        frame 45..85 {
                          n266 = property on="hit block" class="DigNum (strict)"("Val(Sgnl)"=4 ("hit block")) -> ()  [unwired: 2 in, 2 out]
                        }
                        frame 95..135 {
                          n267 = property on="hit block" class="DigNum (strict)"("Val(Sgnl)"=5 ("hit block")) -> ()  [unwired: 2 in, 2 out]
                        }
                      }
                    }
                    frame 285..355 {
                      n268 = case shown="45..85" w520 {
                        frame 0, Default {
                        }
                        frame 45..85 {
                          n269 = property on="hit block" class="DigNum (strict)"("Val(Sgnl)"=6 ("hit block")) -> ()  [unwired: 2 in, 2 out]
                        }
                        frame 95..135 {
                          n270 = property on="hit block" class="DigNum (strict)"("Val(Sgnl)"=7 ("hit block")) -> ()  [unwired: 2 in, 2 out]
                        }
                      }
                    }
                  }
                }
              }
              n271 = case shown="False" w406 {
                tunnel: w405 -> [w464 w491]
                tunnel: [w465 w490] -> w392
                tunnel: w354 -> [w466 w489]
                tunnel: w355 -> [w467 w488]
                frame False {
                  n272 = case shown="250..276" w467 {
                    selector: w467 -> [_ w473]
                    tunnel: w466 -> [_ w478]
                    tunnel: [1 ("f") w477] -> w463
                    frame Default {
                    }
                    frame 250..276 {
                      # "ball size"
                      n273 = property on="Slide" class="Slide (strict)"() -> ("Left"=w487:i32)  [unwired: 2 in, 2 out]
                      n274 = property on="Slide" class="Slide (strict)"() -> ("Top"=w472:i32)  [unwired: 2 in, 2 out]
                      n275 = property on="Slide" class="Slide (strict)"() -> ("Width"=w469:u32)  [unwired: 2 in, 2 out]
                      n276 = Subtract(x=w472, y=w473) -> (x-y=w471:i32)
                      n277 = Subtract(x=w478, y=w487) -> (x-y=w484:i32)
                      n278 = Greater Than 0?(x=w484) -> (x > 0?=w485:bool)
                      n279 = Less?(x=w484, y=w469) -> (x < y?=w486:bool)
                      n280 = Greater?(x=w471, y=3) -> (0:w476:bool)
                      n281 = Less Or Equal?(x=w471, y=6) -> (x <= y?=w475:bool)
                      n282 = And(x=w485, y=w486) -> (x .and. y?=w483:bool)
                      n283 = And(x=w476, y=w475) -> (x .and. y?=w482:bool)
                      n284 = And(x=w483, y=w482) -> (x .and. y?=w481:bool)
                      n285 = Select(t=-1, s=w481, f=1) -> (s? t:f=w477:i32)
                    }
                  }
                  n286 = Multiply(x=w463, y=w464) -> (x*y=w465:i32)
                }
                frame True {
                  n287 = Multiply(x=-1, y=w491) -> (x*y=w490:i32)
                  n288 = case shown="60..130" w489 {
                    tunnel: w488 -> [_ w493 w496 w499 w502]
                    frame 0, Default {
                    }
                    frame 60..130 {
                      n289 = case shown="45..85" w493 {
                        frame 0, Default {
                        }
                        frame 45..85 {
                          n290 = property on="hit block" class="DigNum (strict)"("Val(Sgnl)"=0 ("hit block")) -> ()  [unwired: 2 in, 2 out]
                        }
                        frame 95..135 {
                          n291 = property on="hit block" class="DigNum (strict)"("Val(Sgnl)"=1 ("hit block")) -> ()  [unwired: 2 in, 2 out]
                        }
                      }
                    }
                    frame 135..205 {
                      n292 = case shown="45..85" w496 {
                        frame 0, Default {
                        }
                        frame 45..85 {
                          n293 = property on="hit block" class="DigNum (strict)"("Val(Sgnl)"=2 ("hit block")) -> ()  [unwired: 2 in, 2 out]
                        }
                        frame 95..135 {
                          n294 = property on="hit block" class="DigNum (strict)"("Val(Sgnl)"=3 ("hit block")) -> ()  [unwired: 2 in, 2 out]
                        }
                      }
                    }
                    frame 210..280 {
                      n295 = case shown="45..85" w499 {
                        frame 0, Default {
                        }
                        frame 45..85 {
                          n296 = property on="hit block" class="DigNum (strict)"("Val(Sgnl)"=4 ("hit block")) -> ()  [unwired: 2 in, 2 out]
                        }
                        frame 95..135 {
                          n297 = property on="hit block" class="DigNum (strict)"("Val(Sgnl)"=5 ("hit block")) -> ()  [unwired: 2 in, 2 out]
                        }
                      }
                    }
                    frame 285..355 {
                      n298 = case shown="45..85" w502 {
                        frame 0, Default {
                        }
                        frame 45..85 {
                          n299 = property on="hit block" class="DigNum (strict)"("Val(Sgnl)"=6 ("hit block")) -> ()  [unwired: 2 in, 2 out]
                        }
                        frame 95..135 {
                          n300 = property on="hit block" class="DigNum (strict)"("Val(Sgnl)"=7 ("hit block")) -> ()  [unwired: 2 in, 2 out]
                        }
                      }
                    }
                  }
                }
              }
              n301 = property on="x speed up" class="Str"() -> ("Position"=w375:T5)  [unwired: 2 in, 2 out]
              n302 = property on="y speed up" class="Str"() -> ("Position"=w391:T5)  [unwired: 2 in, 2 out]
              n303 = Unbundle(w375) -> ("Left"=w377:i32, "Top"=w376:i32)
              n304 = Unbundle(w391) -> ("Left"=w384:i32, "Top"=w390:i32)
              n305 = Add(x=w390, y=8) -> (x+y=w388:i32)
              n306 = Add(x=w377, y=8) -> (x+y=w373:i32)
              n307 = Add(x=w380, y=w384) -> (x+y=w383:i32)
              n308 = Add(x=w366, y=w376) -> (x+y=w369:i32)
              n309 = Subtract(x=w354, y=w383) -> (x-y=w382:i32)
              n310 = Subtract(x=w355, y=w369) -> (x-y=w368:i32)
              n311 = Subtract(x=w355, y=w388) -> (x-y=w387:i32)
              n312 = Subtract(x=w354, y=w373) -> (x-y=w372:i32)
              n313 = Absolute Value(x=w382) -> (abs(x)=w381:i32)
              n314 = Absolute Value(x=w387) -> (abs(x)=w386:i32)
              n315 = Absolute Value(x=w368) -> (abs(x)=w367:i32)
              n316 = Absolute Value(x=w372) -> (abs(x)=w371:i32)
              n317 = Less Or Equal?(x=w381, y=w380) -> (x <= y?=w378:bool)
              n318 = Less Or Equal?(x=w386, y=1) -> (x <= y?=w379:bool)
              n319 = Less Or Equal?(x=w367, y=w366) -> (x <= y?=w364:bool)
              n320 = Less Or Equal?(x=w371, y=1) -> (x <= y?=w365:bool)
              n321 = And(x=w378, y=w379) -> (x .and. y?=w361:bool)
              n322 = And(x=w364, y=w365) -> (x .and. y?=w358:bool)
              n323 = Multiply(x=w402, y="x scale") -> (x*y=w403:i32)
              n324 = Multiply(x=w392, y="y scale") -> (x*y=w401:i32)
              n325 = And(x=w359, y=w361) -> (x .and. y?=w360:bool)
              n326 = And(x=w358, y=w356) -> (x .and. y?=w357:bool)
              n327 = Add(x=w403, y=w354) -> (x+y=w349:i32)
              n328 = Add(x=w401, y=w355) -> (x+y=w352:i32)
              n329 = case shown="True" w360 {
                selector: w360 -> [_ w461]
                frame False {
                }
                frame True {
                  n330 = property on="ySpeedUp" class="Bool (strict)"("Val(Sgnl)"=w461) -> ()  [unwired: 2 in, 2 out]
                }
              }
              n331 = case shown="True" w357 {
                selector: w357 -> [_ w460]
                frame False {
                }
                frame True {
                  n332 = property on="xSpeedUp" class="Bool (strict)"("Val(Sgnl)"=w460) -> ()  [unwired: 2 in, 2 out]
                }
              }
              n333 = Select(t=w350, s=w351, f=w349) -> (s? t:f=w348:i32)
              n334 = Select(t=w353, s=w351, f=w352) -> (s? t:f=w347:i32)
              n335 = Greater?(x=w347, y=300) -> (0:w393:bool)
              n336 = Bundle(w348, w347) -> (w397:cluster{i32, i32})  [unwired: 1 in]
              n337 = local read "bricks left"() -> (w398:i32)
              n338 = case shown="True" w393 {
                frame False {
                }
                frame True {
                  n339 = property on="over" class="Bool (strict)"("Val(Sgnl)"=TRUE ("Value (Signaling)")) -> ()  [unwired: 2 in, 2 out]
                }
              }
              n340 = Equal To 0?(x=w398) -> (x = 0?=w395:bool)
              n341 = property on="ball" class="Bool (strict)"("Position"=w397) -> ()  [unwired: 2 in, 2 out]
              n342 = Or(x=w395, y=w393) -> (x .or. y?=w394:bool)
              n343 = Wait Until Next ms Multiple(millisecond multiple=u32 20) -> ()  [unwired: 1 out]
            }
          }
          frame 2 {
            w523 = FALSE
            n344 = local read "ball init pos"() -> (w524:cluster{i32, i32})
            n345 = Random Number (0-1)() -> (number: 0 to 1=w528:dbl)
            n346 = To Long Integer(number=w528) -> (32bit integer=w529:i32)
            n347 = case shown="0, Default" w529 {
              selector: w529 -> [_ w532]
              tunnel: [-1 w532] -> w525
              frame 0, Default {
              }
              frame 1 {
              }
            }
            n348 = Unbundle(w524) -> (w527:i32, w526:i32)
            n349 = while {
              shift-right: [w533] -> _
              shift-left: w527 -> [w541]
              shift-right: [w537] -> _
              shift-left: w526 -> [w540]
              shift-right: [w588] -> _
              shift-left: w525 -> [w593]
              shift-right: [w586] -> _
              shift-left: 1 -> [w591]
              shift-right: [w548] -> _
              shift-left: w523 -> [w545]
              shift-right: [w546] -> _
              shift-left: w523 -> [w543]
              stop <- w581 stop-if-true
              w552 = 45
              w566 = 45
              # "init value set"
              n350 = local read "x hit detec"() -> (w596:bool[][])
              n351 = local read "y hit detec"() -> (w595:bool[][])
              n352 = Not(x=w545) -> (.not. x?=w544:bool)
              n353 = Not(x=w543) -> (.not. x?=w542:bool)
              n354 = flat-sequence {
                tunnel: w541 -> [w602]
                tunnel: w540 -> [w601]
                tunnel: [w600] -> w535
                tunnel: [w599] -> w539
                tunnel: [w598] -> w536
                frame #0 {
                  # "x"
                  # "y"
                  n355 = property on="ball in" class="ColBox"() -> ("Bounds"=w624:T4)  [unwired: 2 in, 2 out]
                  n356 = property on="ball in" class="ColBox"() -> ("Position"=w623:T5)  [unwired: 2 in, 2 out]
                  n357 = Unbundle(w624) -> ("Width"=w607:u32, "Height"=w608:u32)
                  n358 = Unbundle(w623) -> ("Left"=w616:i32, "Top"=w614:i32)
                  n359 = To Quad Integer(1:w608) -> (0:w605:i64)
                  n360 = To Quad Integer(1:w607) -> (0:w606:i64)
                  n361 = Subtract(x=w606, y=u32 10) -> (x-y=w613:i64)
                  n362 = Subtract(x=w605, y=i64 10) -> (x-y=w612:i64)
                  n363 = Subtract(x=w601, y=w614) -> (x-y=w611:i32)
                  n364 = Subtract(x=w602, y=w616) -> (x-y=w615:i32)
                  n365 = Greater?(x=w615, y=-1) -> (0:w621:bool)
                  n366 = Less?(x=w615, y=w613) -> (x < y?=w622:bool)
                  n367 = Greater Or Equal?(x=w611, y=-1) -> (x >= y?=w618:bool)
                  n368 = Less Or Equal?(x=w611, y=w612) -> (x <= y?=w617:bool)
                  n369 = And(x=w621, y=w622) -> (x .and. y?=w620:bool)
                  n370 = And(x=w618, y=w617) -> (x .and. y?=w619:bool)
                  n371 = And(x=w620, y=w619) -> (x .and. y?=w603:bool)
                  n372 = case shown="True" w603 {
                    selector: w603 -> [w625 w628]
                    tunnel: w602 -> [w627 _]
                    tunnel: w601 -> [w626 _]
                    tunnel: [w627 w630] -> w600
                    tunnel: [w626 w629] -> w599
                    tunnel: [w625 w628] -> w598
                    frame False {
                    }
                    frame True {
                      w634 = 2.0 ("y")
                      w641 = 3 ("x")
                      n373 = property on="ball out" class="ColBox"() -> ("Position"=w644:T5)  [unwired: 2 in, 2 out]
                      n374 = Random Number (0-1)() -> (number: 0 to 1=w632:dbl)
                      n375 = Random Number (0-1)() -> (number: 0 to 1=w633:dbl)
                      n376 = Multiply(x=w632, y=w634) -> (x*y=w635:dbl)
                      n377 = Multiply(x=w633, y=w634) -> (x*y=w636:dbl)
                      n378 = Unbundle(w644) -> ("Left"=w643:i32, "Top"=w642:i32)
                      n379 = To Long Integer(number=w635) -> (32bit integer=w638:i32)
                      n380 = To Long Integer(number=w636) -> (32bit integer=w637:i32)
                      n381 = Increment(x=w638) -> (x+1=w639:i32)
                      n382 = Increment(x=w637) -> (x+1=w640:i32)
                      n383 = Add(x=w641, y=w643) -> (x+y=w630:i32)
                      n384 = Add(x=w642, y=w641) -> (x+y=w629:i32)
                      n385 = property on="y scale" class="DigNum (strict)"("Value"=w639) -> ()  [unwired: 2 in, 2 out]
                      n386 = property on="x scale" class="DigNum (strict)"("Value"=w640) -> ()  [unwired: 2 in, 2 out]
                      n387 = Bundle(w630, w629) -> (w645:cluster{i32, i32})  [unwired: 1 in]
                      n388 = property on="ball" class="Bool (strict)"("Position"=w645) -> ()  [unwired: 2 in, 2 out]
                      n389 = Wait (ms)(milliseconds to wait=u32 300) -> ()  [unwired: 1 out]
                    }
                  }
                }
              }
              n390 = Index Array(array=w596, index (row)=w541, index (col)=w540) -> (element=w594:bool)
              n391 = Index Array(array=w595, index (row)=w541, index (col)=w540) -> (element=w592:bool)
              n392 = case shown="True" w594 {
                tunnel: w593 -> [w691 w696]
                tunnel: [w691 w694] -> w588
                tunnel: w541 -> [_ w693]
                tunnel: w540 -> [_ w692]
                frame False {
                }
                frame True {
                  n393 = Multiply(x=-1, y=w696) -> (x*y=w694:i32)
                  n394 = case shown="25..52" w692 {
                    tunnel: w693 -> [_ w697 w700 w703 w706]
                    frame 0, Default {
                    }
                    frame 25..52 {
                      n395 = case shown="318..378" w697 {
                        frame 25..85 {
                          n396 = property on="hit block" class="DigNum (strict)"("Val(Sgnl)"=0 ("hit block")) -> ()  [unwired: 2 in, 2 out]
                        }
                        frame 318..378 {
                          n397 = property on="hit block" class="DigNum (strict)"("Val(Sgnl)"=4 ("hit block")) -> ()  [unwired: 2 in, 2 out]
                        }
                        frame Default {
                        }
                      }
                    }
                    frame 61..88 {
                      n398 = case shown="60..120" w700 {
                        frame 60..120 {
                          n399 = property on="hit block" class="DigNum (strict)"("Val(Sgnl)"=1 ("hit block")) -> ()  [unwired: 2 in, 2 out]
                        }
                        frame 280..340 {
                          n400 = property on="hit block" class="DigNum (strict)"("Val(Sgnl)"=5 ("hit block")) -> ()  [unwired: 2 in, 2 out]
                        }
                        frame Default {
                        }
                      }
                    }
                    frame 97..124 {
                      n401 = case shown="95..155" w703 {
                        frame 95..155 {
                          n402 = property on="hit block" class="DigNum (strict)"("Val(Sgnl)"=2 ("hit block")) -> ()  [unwired: 2 in, 2 out]
                        }
                        frame 245..305 {
                          n403 = property on="hit block" class="DigNum (strict)"("Val(Sgnl)"=6 ("hit block")) -> ()  [unwired: 2 in, 2 out]
                        }
                        frame Default {
                        }
                      }
                    }
                    frame 133..160 {
                      n404 = case shown="60..120" w706 {
                        frame 60..120 {
                          n405 = property on="hit block" class="DigNum (strict)"("Val(Sgnl)"=3 ("hit block")) -> ()  [unwired: 2 in, 2 out]
                        }
                        frame 280..340 {
                          n406 = property on="hit block" class="DigNum (strict)"("Val(Sgnl)"=7 ("hit block")) -> ()  [unwired: 2 in, 2 out]
                        }
                        frame Default {
                        }
                      }
                    }
                  }
                }
              }
              n407 = case shown="False" w592 {
                tunnel: w591 -> [w652 w677]
                tunnel: [w653 w676] -> w586
                tunnel: w541 -> [w650 w674]
                tunnel: w540 -> [w649 w675]
                frame False {
                  n408 = case shown="250..276" w649 {
                    selector: w649 -> [_ w659]
                    tunnel: w650 -> [_ w664]
                    tunnel: [1 ("f") w663] -> w651
                    frame Default {
                    }
                    frame 250..276 {
                      # "ball size"
                      n409 = property on="Slide" class="Slide (strict)"() -> ("Left"=w673:i32)  [unwired: 2 in, 2 out]
                      n410 = property on="Slide" class="Slide (strict)"() -> ("Top"=w658:i32)  [unwired: 2 in, 2 out]
                      n411 = property on="Slide" class="Slide (strict)"() -> ("Width"=w655:u32)  [unwired: 2 in, 2 out]
                      n412 = Subtract(x=w658, y=w659) -> (x-y=w657:i32)
                      n413 = Subtract(x=w664, y=w673) -> (x-y=w670:i32)
                      n414 = Greater Than 0?(x=w670) -> (x > 0?=w671:bool)
                      n415 = Less?(x=w670, y=w655) -> (x < y?=w672:bool)
                      n416 = Greater?(x=w657, y=3) -> (0:w662:bool)
                      n417 = Less Or Equal?(x=w657, y=6) -> (x <= y?=w661:bool)
                      n418 = And(x=w671, y=w672) -> (x .and. y?=w669:bool)
                      n419 = And(x=w662, y=w661) -> (x .and. y?=w668:bool)
                      n420 = And(x=w669, y=w668) -> (x .and. y?=w667:bool)
                      n421 = Select(t=-1, s=w667, f=1) -> (s? t:f=w663:i32)
                    }
                  }
                  n422 = Multiply(x=w651, y=w652) -> (x*y=w653:i32)
                }
                frame True {
                  n423 = Multiply(x=-1, y=w677) -> (x*y=w676:i32)
                  n424 = case shown="133..160" w675 {
                    tunnel: w674 -> [_ w679 w682 w685 w688]
                    frame 0, Default {
                    }
                    frame 25..52 {
                      n425 = case shown="25..85" w679 {
                        frame 25..85 {
                          n426 = property on="hit block" class="DigNum (strict)"("Val(Sgnl)"=0 ("hit block")) -> ()  [unwired: 2 in, 2 out]
                        }
                        frame 318..378 {
                          n427 = property on="hit block" class="DigNum (strict)"("Val(Sgnl)"=4 ("hit block")) -> ()  [unwired: 2 in, 2 out]
                        }
                        frame Default {
                        }
                      }
                    }
                    frame 61..88 {
                      n428 = case shown="60..120" w682 {
                        frame 60..120 {
                          n429 = property on="hit block" class="DigNum (strict)"("Val(Sgnl)"=1 ("hit block")) -> ()  [unwired: 2 in, 2 out]
                        }
                        frame 280..340 {
                          n430 = property on="hit block" class="DigNum (strict)"("Val(Sgnl)"=5 ("hit block")) -> ()  [unwired: 2 in, 2 out]
                        }
                        frame Default {
                        }
                      }
                    }
                    frame 97..124 {
                      n431 = case shown="95..155" w685 {
                        frame 95..155 {
                          n432 = property on="hit block" class="DigNum (strict)"("Val(Sgnl)"=2 ("hit block")) -> ()  [unwired: 2 in, 2 out]
                        }
                        frame 245..305 {
                          n433 = property on="hit block" class="DigNum (strict)"("Val(Sgnl)"=6 ("hit block")) -> ()  [unwired: 2 in, 2 out]
                        }
                        frame Default {
                        }
                      }
                    }
                    frame 133..160 {
                      n434 = case shown="60..120" w688 {
                        frame 60..120 {
                          n435 = property on="hit block" class="DigNum (strict)"("Val(Sgnl)"=3 ("hit block")) -> ()  [unwired: 2 in, 2 out]
                        }
                        frame 280..340 {
                          n436 = property on="hit block" class="DigNum (strict)"("Val(Sgnl)"=7 ("hit block")) -> ()  [unwired: 2 in, 2 out]
                        }
                        frame Default {
                        }
                      }
                    }
                  }
                }
              }
              n437 = property on="x speed up" class="Str"() -> ("Position"=w561:T5)  [unwired: 2 in, 2 out]
              n438 = property on="y speed up" class="Str"() -> ("Position"=w577:T5)  [unwired: 2 in, 2 out]
              n439 = Unbundle(w561) -> ("Left"=w563:i32, "Top"=w562:i32)
              n440 = Unbundle(w577) -> ("Left"=w570:i32, "Top"=w576:i32)
              n441 = Add(x=w576, y=8) -> (x+y=w574:i32)
              n442 = Add(x=w563, y=8) -> (x+y=w559:i32)
              n443 = Add(x=w566, y=w570) -> (x+y=w569:i32)
              n444 = Add(x=w552, y=w562) -> (x+y=w555:i32)
              n445 = Subtract(x=w541, y=w569) -> (x-y=w568:i32)
              n446 = Subtract(x=w540, y=w555) -> (x-y=w554:i32)
              n447 = Subtract(x=w540, y=w574) -> (x-y=w573:i32)
              n448 = Subtract(x=w541, y=w559) -> (x-y=w558:i32)
              n449 = local read "x scale"() -> (w579:i32)
              n450 = local read "y scale"() -> (w578:i32)
              n451 = Absolute Value(x=w568) -> (abs(x)=w567:i32)
              n452 = Absolute Value(x=w573) -> (abs(x)=w572:i32)
              n453 = Absolute Value(x=w554) -> (abs(x)=w553:i32)
              n454 = Absolute Value(x=w558) -> (abs(x)=w557:i32)
              n455 = Less Or Equal?(x=w567, y=w566) -> (x <= y?=w564:bool)
              n456 = Less Or Equal?(x=w572, y=1) -> (x <= y?=w565:bool)
              n457 = Less Or Equal?(x=w553, y=w552) -> (x <= y?=w550:bool)
              n458 = Less Or Equal?(x=w557, y=1) -> (x <= y?=w551:bool)
              n459 = Multiply(x=w588, y=w579) -> (x*y=w589:i32)
              n460 = Multiply(x=w586, y=w578) -> (x*y=w587:i32)
              n461 = And(x=w564, y=w565) -> (x .and. y?=w549:bool)
              n462 = And(x=w550, y=w551) -> (x .and. y?=w547:bool)
              n463 = Add(x=w589, y=w541) -> (x+y=w534:i32)
              n464 = Add(x=w587, y=w540) -> (x+y=w538:i32)
              n465 = And(x=w544, y=w549) -> (x .and. y?=w548:bool)
              n466 = And(x=w547, y=w542) -> (x .and. y?=w546:bool)
              n467 = Select(t=w535, s=w536, f=w534) -> (s? t:f=w533:i32)
              n468 = case shown="True" w548 {
                selector: w548 -> [_ w647]
                frame False {
                }
                frame True {
                  n469 = property on="ySpeedUp" class="Bool (strict)"("Val(Sgnl)"=w647) -> ()  [unwired: 2 in, 2 out]
                }
              }
              n470 = Select(t=w539, s=w536, f=w538) -> (s? t:f=w537:i32)
              n471 = case shown="True" w546 {
                selector: w546 -> [_ w646]
                frame False {
                }
                frame True {
                  n472 = property on="xSpeedUp" class="Bool (strict)"("Val(Sgnl)"=w646) -> ()  [unwired: 2 in, 2 out]
                }
              }
              n473 = Greater?(x=w537, y=300) -> (0:w580:bool)
              n474 = Bundle(w533, w537) -> (w584:cluster{i32, i32})  [unwired: 1 in]
              n475 = local read "bricks left"() -> (w585:i32)
              n476 = case shown="True" w580 {
                frame False {
                }
                frame True {
                  n477 = property on="over" class="Bool (strict)"("Val(Sgnl)"=TRUE ("Value (Signaling)")) -> ()  [unwired: 2 in, 2 out]
                }
              }
              n478 = property on="ball" class="Bool (strict)"("Position"=w584) -> ()  [unwired: 2 in, 2 out]
              n479 = Equal To 0?(x=w585) -> (x = 0?=w582:bool)
              n480 = Or(x=w582, y=w580) -> (x .or. y?=w581:bool)
              n481 = Wait Until Next ms Multiple(millisecond multiple=u32 20) -> ()  [unwired: 1 out]
            }
          }
        }
        n482 = local write "game states"(T1."End" ("game states")) -> ()
        n483 = while {
          stop <- w777 stop-if-true
          n484 = event shown="[2] \"bricks left\": Value Change" {
            selector: _ -> [_ _ _ _]
            dyn-events: _ -> [_ _ _ _]
            timeout: _ -> [_ _ _ _]
            tunnel: [_ _ w841 w843] -> w777
            event Key Down {
              n485 = event-data() -> ("VKey"=w780:T6)  [unwired: 1 in]
              n486 = case shown="\"Up\"" w780 {
                tunnel: 40 -> [_ _ _ w796 w808]
                tunnel: 4 ("y") -> [_ _ _ w794 w806]
                frame "ASCII", Default {
                }
                frame "Up" {
                  n487 = property on="Slide" class="Slide (strict)"() -> ("Top"=w782:i32)  [unwired: 2 in, 2 out]
                  n488 = Equal?(x=w782, y=275) -> (x = y?=w783:bool)
                  n489 = case shown="True" w783 {
                    tunnel: w782 -> [_ _]
                    frame False {
                    }
                    frame True {
                      n490 = for {
                        N: 5 -> [_]
                        n491 = property on="Slide" class="Slide (strict)"() -> ("Top"=w785:i32)  [unwired: 2 in, 2 out]
                        n492 = Subtract(x=w785, y=2) -> (x-y=w786:i32)
                        n493 = property on="Slide" class="Slide (strict)"("Top"=w786) -> ()  [unwired: 2 in, 2 out]
                      }
                    }
                  }
                }
                frame "Down" {
                  n494 = property on="Slide" class="Slide (strict)"() -> ("Top"=w789:i32)  [unwired: 2 in, 2 out]
                  n495 = Equal?(x=w789, y=265) -> (x = y?=w790:bool)
                  n496 = case shown="True" w790 {
                    tunnel: w789 -> [_ w791]
                    frame False {
                    }
                    frame True {
                      n497 = Add(x=w791, y=10) -> (x+y=w792:i32)
                      n498 = property on="Slide" class="Slide (strict)"("Top"=w792) -> ()  [unwired: 2 in, 2 out]
                    }
                  }
                }
                frame "Left" {
                  n499 = property on="Slide" class="Slide (strict)"() -> ("Left"=w797:i32)  [unwired: 2 in, 2 out]
                  n500 = Quotient & Remainder(x=w796, y=w794) -> (floor(x/y)=w795:i32)  [unwired: 1 out]
                  n501 = Greater?(x=w797, y=w796) -> (0:w798:bool)
                  n502 = case shown="True" w798 {
                    tunnel: w797 -> [_ w802]
                    tunnel: w795 -> [_ w801]
                    tunnel: w794 -> [_ w800]
                    frame False {
                      n503 = property on="Slide" class="Slide (strict)"("Left"=0 ("Position:Left")) -> ()  [unwired: 2 in, 2 out]
                    }
                    frame True {
                      n504 = for {
                        N: w800 -> [_]
                        tunnel: w802 -> [_]
                        tunnel: w801 -> [w804]
                        n505 = property on="Slide" class="Slide (strict)"() -> ("Left"=w803:i32)  [unwired: 2 in, 2 out]
                        n506 = Subtract(x=w803, y=w804) -> (x-y=w805:i32)
                        n507 = property on="Slide" class="Slide (strict)"("Left"=w805) -> ()  [unwired: 2 in, 2 out]
                      }
                    }
                  }
                }
                frame "Right" {
                  n508 = property on="Slide" class="Slide (strict)"() -> ("Left"=w813:i32, "Width"=w810:u32)  [unwired: 2 in, 2 out]
                  n509 = Subtract(x=405, y=w810) -> (x-y=w809:u32)
                  n510 = Subtract(x=w809, y=w808) -> (x-y=w811:u32)
                  n511 = Quotient & Remainder(x=w808, y=w806) -> (floor(x/y)=w807:i32)  [unwired: 1 out]
                  n512 = Less?(x=w813, y=w811) -> (x < y?=w814:bool)
                  n513 = case shown="True" w814 {
                    tunnel: w813 -> [_ _]
                    tunnel: w809 -> [w815 _]
                    tunnel: w807 -> [_ w817]
                    tunnel: w806 -> [_ w816]
                    frame False {
                      n514 = property on="Slide" class="Slide (strict)"("Left"=w815) -> ()  [unwired: 2 in, 2 out]
                    }
                    frame True {
                      n515 = for {
                        N: w816 -> [_]
                        tunnel: w817 -> [w819]
                        n516 = property on="Slide" class="Slide (strict)"() -> ("Left"=w818:i32)  [unwired: 2 in, 2 out]
                        n517 = Add(x=w818, y=w819) -> (x+y=w820:i32)
                        n518 = property on="Slide" class="Slide (strict)"("Left"=w820) -> ()  [unwired: 2 in, 2 out]
                      }
                    }
                  }
                }
              }
            }
            event Key Repeat {
              n519 = event-data() -> ("VKey"=w822:T6)  [unwired: 1 in]
              n520 = case shown="\"Right\"" w822 {
                tunnel: 10 -> [_ w823 w830]
                frame "ASCII", Default {
                }
                frame "Left" {
                  n521 = property on="Slide" class="Slide (strict)"() -> ("Left"=w824:i32)  [unwired: 2 in, 2 out]
                  n522 = Greater?(x=w824, y=w823) -> (0:w825:bool)
                  n523 = case shown="False" w825 {
                    tunnel: w824 -> [_ w828]
                    tunnel: w823 -> [_ w827]
                    frame False {
                      n524 = property on="Slide" class="Slide (strict)"("Left"=0 ("Position:Left")) -> ()  [unwired: 2 in, 2 out]
                    }
                    frame True {
                      n525 = Subtract(x=w828, y=w827) -> (x-y=w829:i32)
                      n526 = property on="Slide" class="Slide (strict)"("Left"=w829) -> ()  [unwired: 2 in, 2 out]
                    }
                  }
                }
                frame "Right" {
                  n527 = property on="Slide" class="Slide (strict)"() -> ("Left"=w835:i32, "Width"=w833:u32)  [unwired: 2 in, 2 out]
                  n528 = Subtract(x=405, y=w833) -> (x-y=w831:u32)
                  n529 = Subtract(x=w831, y=w830) -> (x-y=w832:u32)
                  n530 = Less?(x=w835, y=w832) -> (x < y?=w836:bool)
                  n531 = case shown="True" w836 {
                    tunnel: w835 -> [_ w840]
                    tunnel: w831 -> [w837 _]
                    tunnel: w830 -> [_ w838]
                    frame False {
                      n532 = property on="Slide" class="Slide (strict)"("Left"=w837) -> ()  [unwired: 2 in, 2 out]
                    }
                    frame True {
                      n533 = Add(x=w840, y=w838) -> (x+y=w839:i32)
                      n534 = property on="Slide" class="Slide (strict)"("Left"=w839) -> ()  [unwired: 2 in, 2 out]
                    }
                  }
                }
              }
            }
            event "bricks left": Value Change {
              n535 = event-data() -> ("NewVal"=w842:i32)  [unwired: 1 in]
              n536 = Equal To 0?(x=w842) -> (x = 0?=w841:bool)
            }
            event "over": Value Change {
              n537 = event-data() -> ("NewVal"=w843:bool)  [unwired: 1 in]
            }
          }
        }
        n538 = local read "Level"() -> (w271:i32)
        n539 = while {
          stop <- w319 stop-if-true
          n540 = event shown="[0] \"ySpeedUp\": Value Change" {
            selector: _ -> [_ _ _ _]
            dyn-events: _ -> [_ _ _ _]
            timeout: _ -> [_ _ _ _]
            tunnel: [_ _ w334 w335] -> w319
            event "ySpeedUp": Value Change {
              n541 = event-data() -> ("NewVal"=w321:bool)  [unwired: 1 in]
              n542 = local read "y scale"() -> (w320:i32)
              n543 = Less?(x=w320, y=3) -> (x < y?=w322:bool)
              n544 = And(x=w322, y=w321) -> (x .and. y?=w323:bool)
              n545 = case shown="False" w323 {
                tunnel: w320 -> [_ w326]
                frame False {
                }
                frame True {
                  n546 = Increment(x=w326) -> (x+1=w325:i32)
                  n547 = local write "y scale"(w325) -> ()
                }
              }
            }
            event "xSpeedUp": Value Change {
              n548 = event-data() -> ("NewVal"=w327:bool)  [unwired: 1 in]
              n549 = local read "x scale"() -> (w328:i32)
              n550 = Less?(x=w328, y=3) -> (x < y?=w329:bool)
              n551 = And(x=w329, y=w327) -> (x .and. y?=w330:bool)
              n552 = case shown="True" w330 {
                tunnel: w328 -> [_ w333]
                frame False {
                }
                frame True {
                  n553 = Increment(x=w333) -> (x+1=w332:i32)
                  n554 = local write "x scale"(w332) -> ()
                }
              }
            }
            event "over": Value Change {
              n555 = event-data() -> ("NewVal"=w334:bool)  [unwired: 1 in]
            }
            event "bricks left": Value Change {
              n556 = event-data() -> ("NewVal"=w336:i32)  [unwired: 1 in]
              n557 = Equal To 0?(x=w336) -> (x = 0?=w335:bool)
            }
          }
        }
        n558 = case shown="2" w271 {
          tunnel: [0 30] -> w270
          frame 0, Default {
          }
          frame 2 {
          }
        }
        n559 = while {
          shift-right: [w278] -> _
          shift-left: 0 -> [w279]
          tunnel: w270 -> [w277]
          stop <- w280 stop-if-true
          n560 = event shown="[0] Timeout" {
            selector: _ -> [_ _ _]
            dyn-events: _ -> [_ _ _]
            timeout: u32 1 ("millisecond multiple") -> [_ _ _]
            tunnel: w279 -> [w283 w314 w316]
            tunnel: [_ w315 w317] -> w280
            tunnel: [w285 w314 w316] -> w278
            tunnel: w277 -> [w282 _ _]
            event Timeout {
              n561 = event-data() -> ()  [unwired: 1 in, 1 out]
              n562 = property on="ball in" class="ColBox"() -> ("Left"=w287:i32)  [unwired: 2 in, 2 out]
              n563 = Quotient & Remainder(x=w283, y=8) -> (x-y*floor(x/y)=w289:i32)  [unwired: 1 out]
              n564 = case shown="7" w289 {
                tunnel: w287 -> [w292 w295 w298 w301 w304 w307 w310 w313]
                tunnel: [w291 w294 w297 w300 w303 w306 w309 w312] -> w286
                tunnel: w282 -> [w290 w293 w296 w299 w302 w305 w308 w311]
                frame 0, Default {
                  n565 = Add(x=w292, y=w290) -> (x+y=w291:i32)
                }
                frame 1 {
                  n566 = Add(x=w295, y=w293) -> (x+y=w294:i32)
                }
                frame 2 {
                  n567 = Subtract(x=w298, y=w296) -> (x-y=w297:i32)
                }
                frame 3 {
                  n568 = Subtract(x=w301, y=w299) -> (x-y=w300:i32)
                }
                frame 4 {
                  n569 = Subtract(x=w304, y=w302) -> (x-y=w303:i32)
                }
                frame 5 {
                  n570 = Subtract(x=w307, y=w305) -> (x-y=w306:i32)
                }
                frame 6 {
                  n571 = Add(x=w310, y=w308) -> (x+y=w309:i32)
                }
                frame 7 {
                  n572 = Add(x=w313, y=w311) -> (x+y=w312:i32)
                }
              }
              n573 = Increment(x=w283) -> (x+1=w285:i32)
              n574 = Wait (ms)(milliseconds to wait=u32 1000) -> ()  [unwired: 1 out]
              n575 = property on="ball in" class="ColBox"("Left"=w286) -> ()  [unwired: 2 in, 2 out]
            }
            event "over": Value Change {
              n576 = event-data() -> ("NewVal"=w315:bool)  [unwired: 1 in]
            }
            event "bricks left": Value Change {
              n577 = event-data() -> ("NewVal"=w318:i32)  [unwired: 1 in]
              n578 = Equal To 0?(x=w318) -> (x = 0?=w317:bool)
            }
          }
        }
      }
      frame "End" {
        w844 = FALSE ("Visible")
        n579 = local read "start timer"() -> (w853:u32)
        n580 = Tick Count (ms)() -> (millisecond timer value=w854:u32)
        n581 = local read "bricks left"() -> (w848:i32)
        n582 = Subtract(x=w854, y=w853) -> (x-y=w852:u32)
        n583 = local read "Level"() -> (w859:i32)
        n584 = Quotient & Remainder(x=w852, y=u32 10) -> (floor(x/y)=w850:u32)  [unwired: 1 out]
        n585 = local read "bricks left"() -> (w857:i32)
        n586 = Wait (ms)(milliseconds to wait=u32 1000) -> ()  [unwired: 1 out]
        n587 = Equal To 0?(x=w848) -> (x = 0?=w847:bool)
        n588 = local read "Score"() -> (w856:i32)
        n589 = Divide(x=w850, y=u32 100) -> (x/y=w858:dbl)
        n590 = case shown="1, Default" w859 {
          tunnel: [w881 w894] -> w845
          tunnel: w847 -> [w880 w893]
          frame 1, Default {
            n591 = case shown="True" w880 {
              tunnel: [TRUE FALSE] -> w881
              frame False {
                n592 = Wait (ms)(milliseconds to wait=u32 2000) -> ()  [unwired: 1 out]
                n593 = property on="game string" class="Str"("Visible"=TRUE, "Value"="Game Over", "DisabledEnum"=T3."Disabled" ("Disabled")) -> ()  [unwired: 2 in, 2 out]
              }
              frame True {
                n594 = local write "game states"(T1."Initialize" ("game states")) -> ()
                n595 = property on="game string" class="Str"("Visible"=TRUE, "Value"="Next Level", "DisabledEnum"=T3."Disabled" ("Disabled")) -> ()  [unwired: 2 in, 2 out]
                n596 = local write "Level"(2 ("Level")) -> ()
              }
            }
          }
          frame 2 {
            n597 = case shown="True" w893 {
              tunnel: [TRUE TRUE] -> w894
              frame False {
                n598 = Wait (ms)(milliseconds to wait=u32 2000) -> ()  [unwired: 1 out]
                n599 = property on="game string" class="Str"("Visible"=TRUE, "Value"="Game Over", "DisabledEnum"=T3."Disabled" ("Disabled")) -> ()  [unwired: 2 in, 2 out]
              }
              frame True {
                n600 = Wait (ms)(milliseconds to wait=u32 2000) -> ()  [unwired: 1 out]
                n601 = property on="game string" class="Str"("Visible"=TRUE, "Value"="Congratulations !", "DisabledEnum"=T3."Disabled" ("Disabled")) -> ()  [unwired: 2 in, 2 out]
              }
            }
          }
        }
        n602 = case shown="1, Default" w857 {
          selector: w857 -> [_ w878]
          tunnel: [w864 w874] -> w855
          tunnel: w856 -> [w861 w873]
          tunnel: w858 -> [w860 _]
          frame 0 {
            n603 = Logarithm Base 2(1:w860) -> (0:w872:dbl)
            n604 = Subtract(x=10.0, y=w872) -> (x-y=w870:dbl)
            n605 = Multiply(x=w870, y=1000.0) -> (x*y=w868:dbl)
            n606 = To Long Integer(number=w868) -> (32bit integer=w866:i32)
            n607 = Greater Than 0?(x=w866) -> (x > 0?=w867:bool)
            n608 = Select(t=w866, s=w867, f=0) -> (s? t:f=w863:i32)
            n609 = Compound Arithmetic op=ADD(w863, 10000, w861) -> (w864:i32)
          }
          frame 1, Default {
            n610 = Subtract(x=8, y=w878) -> (x-y=w877:i32)
            n611 = Multiply(x=1000, y=w877) -> (x*y=w875:i32)
            n612 = Add(x=w875, y=w873) -> (x+y=w874:i32)
          }
        }
        n613 = property on="y speed up" class="Str"("Visible"=w844) -> ()  [unwired: 2 in, 2 out]
        n614 = property on="x speed up" class="Str"("Visible"=w844) -> ()  [unwired: 2 in, 2 out]
        n615 = property on="ball in" class="ColBox"("Visible"=w844) -> ()  [unwired: 2 in, 2 out]
        n616 = property on="ball out" class="ColBox"("Visible"=w844) -> ()  [unwired: 2 in, 2 out]
        n617 = local write "Score"(w855) -> ()
      }
    }
  }
  "Score" <- 0 ("Score")
  "y speed up" <- "◆□◆□◆□" ("x speed up")
  "x speed up" <- "■\n△\n■\n△\n△" ("y speed up")
